vi "THzTime_SPEED_control_2_points_scan_TA_170302.vi"(1 "ESP300 Axis":i8=1, 2 "ESP300 Address":string="1", 4 "Lockin Address":string="12") -> ()   [LabVIEW 2010]
panel:
  out "Current Round":i32
  in  "ESP300 Axis 2":i8=2
  in  "Delay (ms)":u32=10000
  in  "# of Round":i8=10
  in  "Position 2":sgl=-33.5 min=-75 max=75 format="%#.3f"
  in  "Position 1":sgl=-35.0 min=-75 max=75 format="%#.3f"
  out "Y position":dbl=-149.05 format="%#.3p"
  out "X position":dbl=857.9 format="%#.3p"
  out "Power meter":dbl=68.74000000000001 format="%#.3p"
  in  "Save File Name":string
  in  "Launch server?":bool
  in  "Authorize?":bool=TRUE
  in  "CONEX-PSD9 Instrument Key 2":string="CONEX-PSD (A6ULD73M)"
  in  "Interdelay (ms)":dbl=20.0
  in  "pre delay(ms)":dbl=300.0
  out "Lock-in Y-Channel":dbl=2.5466e-11 format="%#.3p"
  out "Lock-in X-Channel":dbl=-5.457e-12 format="%#.3p"
  out "THz Time-domain Signal Wave":cluster{"x-axis":sgl[], "y-axis":dbl[]}(graph)={"x-axis"=[-3.0, -2.99, -2.98, -2.97, -2.96, -2.95, -2.94, -2.93, -2.92, -2.91, -2.9, -2.89, -2.88, -2.87, -2.86, -2.85, -2.84, -2.83, -2.82, -2.81, -2.8, -2.79, -2.78, -2.77, -2.76, -2.75, -2.74, -2.73, -2.72, -2.71, -2.7, -2.69, -2.68, -2.67, -2.66, -2.65, -2.64, -2.63, -2.6200001, -2.61, -2.6, -2.59, -2.58, -2.57, -2.56, -2.55, -2.54, -2.53, -2.52, -2.51, -2.5, -2.49, -2.48, -2.47, -2.46, -2.45, -2.44, -2.43, -2.42, -2.41, -2.4, -2.39, -2.38, -2.3700001, -2.3600001, -2.35, -2.34, -2.33, -2.32, -2.31, -2.3, -2.29, -2.28, -2.27, -2.26, -2.25, -2.24, -2.23, -2.22, -2.21, -2.2, -2.19, -2.18, -2.17, -2.16, -2.15, -2.14, -2.13, -2.1200001, -2.1100001, -2.1, -2.09, -2.08, -2.07, -2.06, -2.05, -2.04, -2.03, -2.02, -2.01, -2.0, -1.99, -1.98, -1.97, -1.96, -1.95, -1.94, -1.9300001, -1.9200001, -1.91, -1.9, -1.89, -1.88, -1.87, -1.86, -1.85, -1.84, -1.83, -1.82, -1.8100001, -1.8000001, -1.7900001, -1.78, -1.77, -1.76, -1.75, -1.74, -1.73, -1.72, -1.71, -1.7, -1.69, -1.6800001, -1.6700001, -1.6600001, -1.65, -1.64, -1.63, -1.62, -1.61, -1.6, -1.59, -1.58, -1.57, -1.5600001, -1.5500001, -1.5400001, -1.5300001, -1.52, -1.51, -1.5, -1.49, -1.48, -1.47, -1.46, -1.45, -1.44, -1.4300001, -1.4200001, -1.4100001, -1.4000001, -1.39, -1.38, -1.37, -1.36, -1.35, -1.34, -1.33, -1.32, -1.3100001, -1.3000001, -1.2900001, -1.2800001, -1.27, -1.26, -1.25, -1.24, -1.23, -1.22, -1.21, -1.2, -1.19, -1.1800001, -1.1700001, -1.1600001, -1.1500001, -1.14, -1.13, -1.12, -1.11, -1.1, -1.09, -1.08, -1.07, -1.0600001, -1.0500001, -1.0400001, -1.0300001, -1.0200001, -1.01, -1.0, -0.99000007], "y-axis"=[6.18461e-11, 6.18461e-11, 6.275559999999999e-11, 6.457460000000001e-11, 6.54841e-11, 6.63936e-11, 6.821255e-11, 7.00315e-11, 7.18505e-11, 7.36695e-11, 7.54885e-11, 7.6398e-11, 7.6398e-11, 7.8217e-11, 7.8217e-11, 7.8217e-11, 7.8217e-11, 7.8217e-11, 7.8217e-11, 7.8217e-11, 7.8217e-11, 7.8217e-11, 7.8217e-11, 7.8217e-11, 7.73075e-11, 7.6398e-11, 7.54885e-11, 7.4579e-11, 7.4579e-11, 7.4579e-11, 7.4579e-11, 7.4579e-11, 7.4579e-11, 7.4579e-11, 7.36695e-11, 7.276e-11, 7.276e-11, 7.276e-11, 7.18505e-11, 7.18505e-11, 7.276e-11, 7.18505e-11, 7.0941e-11, 7.0941e-11, 7.00315e-11, 6.9122e-11, 6.821255e-11, 6.63936e-11, 6.457460000000001e-11, 6.275559999999999e-11, 6.18461e-11, 6.18461e-11, 6.275559999999999e-11, 6.36651e-11, 6.63936e-11, 6.912205e-11, 7.275999999999999e-11, 7.6398e-11, 7.91265e-11, 8.09455e-11, 8.27645e-11, 8.3674e-11, 8.3674e-11, 8.3674e-11, 8.27645e-11, 8.09455e-11, 7.821699999999999e-11, 7.36695e-11, 6.821255e-11, 6.09366e-11, 5.54795e-11, 4.911295e-11, 4.2746500000000003e-11, 3.7289500000000003e-11, 3.2742e-11, 3.001355e-11, 2.7285e-11, 2.7285e-11, 2.819455e-11, 3.092305e-11, 3.4561000000000003e-11, 3.7289500000000003e-11, 3.9108499999999995e-11, 4.09275e-11, 4.45655e-11, 4.638445e-11, 5.00224e-11, 5.18414e-11, 5.36604e-11, 5.72985e-11, 5.82081e-11, 5.82081e-11, 5.82081e-11, 6.00271e-11, 6.09366e-11, 6.275559999999999e-11, 6.457460000000001e-11, 6.730305e-11, 7.00315e-11, 7.18505e-11, 7.36695e-11, 7.54885e-11, 7.6398e-11, 7.73075e-11, 7.8217e-11, 7.8217e-11, 7.8217e-11, 7.8217e-11, 7.8217e-11, 7.8217e-11, 7.8217e-11, 7.8217e-11, 7.8217e-11, 7.8217e-11, 7.8217e-11, 7.8217e-11, 7.91265e-11, 8.0036e-11, 8.0036e-11, 7.91265e-11, 7.8217e-11, 7.8217e-11, 7.8217e-11, 7.8217e-11, 7.91265e-11, 8.0036e-11, 8.0036e-11, 8.0036e-11, 8.09455e-11, 8.1855e-11, 8.09455e-11, 8.0036e-11, 7.91265e-11, 7.8217e-11, 7.8217e-11, 7.73075e-11, 7.54885e-11, 7.36695e-11, 7.18505e-11, 6.9122e-11, 6.73031e-11, 6.54841e-11, 6.457460000000001e-11, 6.36651e-11, 6.275559999999999e-11, 6.09366e-11, 6.00271e-11, 6.00271e-11, 6.00271e-11, 6.00271e-11, 6.09366e-11, 6.18461e-11, 6.18461e-11, 6.18461e-11, 6.275559999999999e-11, 6.36651e-11, 6.457460000000001e-11, 6.54841e-11, 6.457460000000001e-11, 6.36651e-11, 6.36651e-11, 6.36651e-11, 6.36651e-11, 6.36651e-11, 6.36651e-11, 6.36651e-11, 6.36651e-11, 6.36651e-11, 6.36651e-11, 6.36651e-11, 6.36651e-11, 6.36651e-11, 6.457460000000001e-11, 6.54841e-11, 6.457460000000001e-11, 6.457460000000001e-11, 6.54841e-11, 6.63936e-11, 6.73031e-11, 6.73031e-11, 6.9122e-11, 6.73031e-11, 6.821255e-11, 6.9122e-11, 6.9122e-11, 6.73031e-11, 6.821255e-11, 6.9122e-11, 6.9122e-11, 6.9122e-11, 6.9122e-11, 6.821255e-11, 6.73031e-11, 6.73031e-11, 6.73031e-11, 6.73031e-11, 6.73031e-11, 6.73031e-11, 6.63936e-11, 6.63936e-11, 6.54841e-11, 6.54841e-11]}
  in  "Autosave Directory for Long-term Average Scan":path=path "D:/taianh/Measurement Data"
  in  "OK Button":bool
  out "Data Type":string="outp ? 1"
  in  "Enum":enum16{"X", "Y", "Abs"}(ring)
  in  "Draw":bool
  in  "Exit Program":bool
  in  "Short term \nAverage#":i8=1
  in  "Step":sgl=0.005 min=0 max=10000 format="%.3f"
  in  "End Position":sgl=-10.5 min=-75 max=75 format="%#.3f"
  in  "Start Position":sgl=-6.0 min=-75 max=75 format="%#.3f"
  # "THz Experiment"
  # "Data"
  # "Auto-offset"
  # "Start Position (mm)"
  # "End Position (mm)"
  # "Step (mm)"
  # "Point Avg"
  # "Number of Round"
  # "Position 1 (mm)"
  # "Position 2 (mm)"
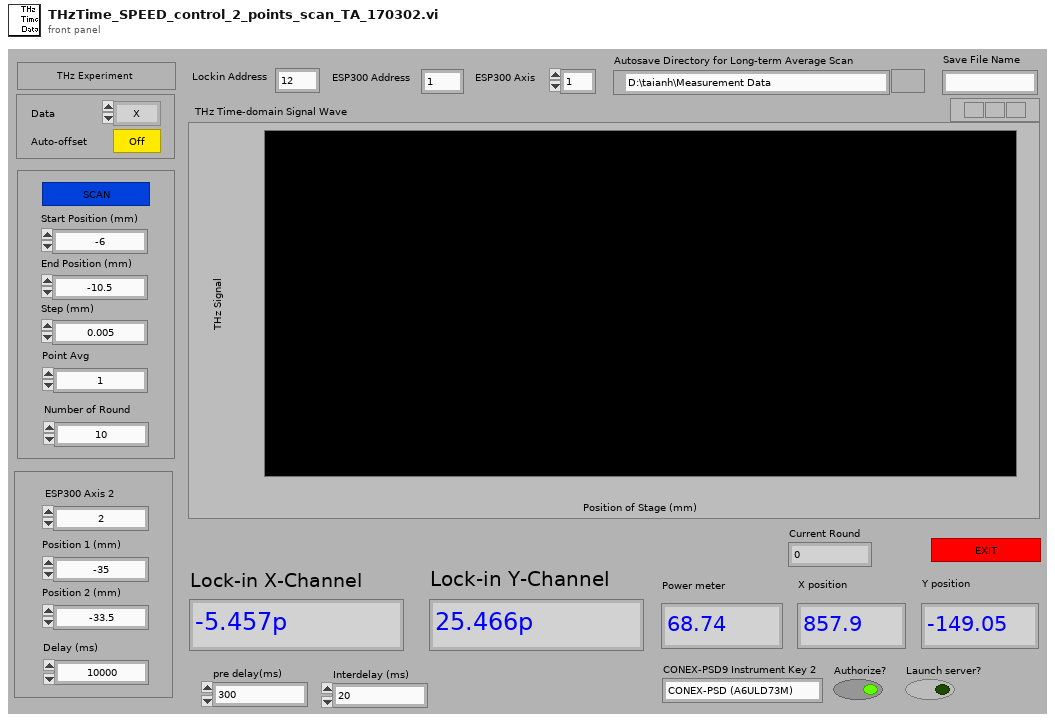
[diagram p1: front panel]
types:
  T1 = cluster{"ConexPSD Reference":refnum<k24>, "error out":errorcluster, "Component ID":i32}
  T2 = cluster{"Step Number":i32, "Step":sgl, "Start Position":sgl, "Time-out":i32, "Lockin Address":string, "Short term \nAverage#":i8, i32, "ESP300 Axis":i8, "Value":string, "pre delay(ms)":dbl, "Interdelay (ms)":dbl, "Autosave Directory for Long-term Average Scan":path, cluster{"ConexPSD Reference":refnum<k24>, "error out":errorcluster, "Component ID":i32}}
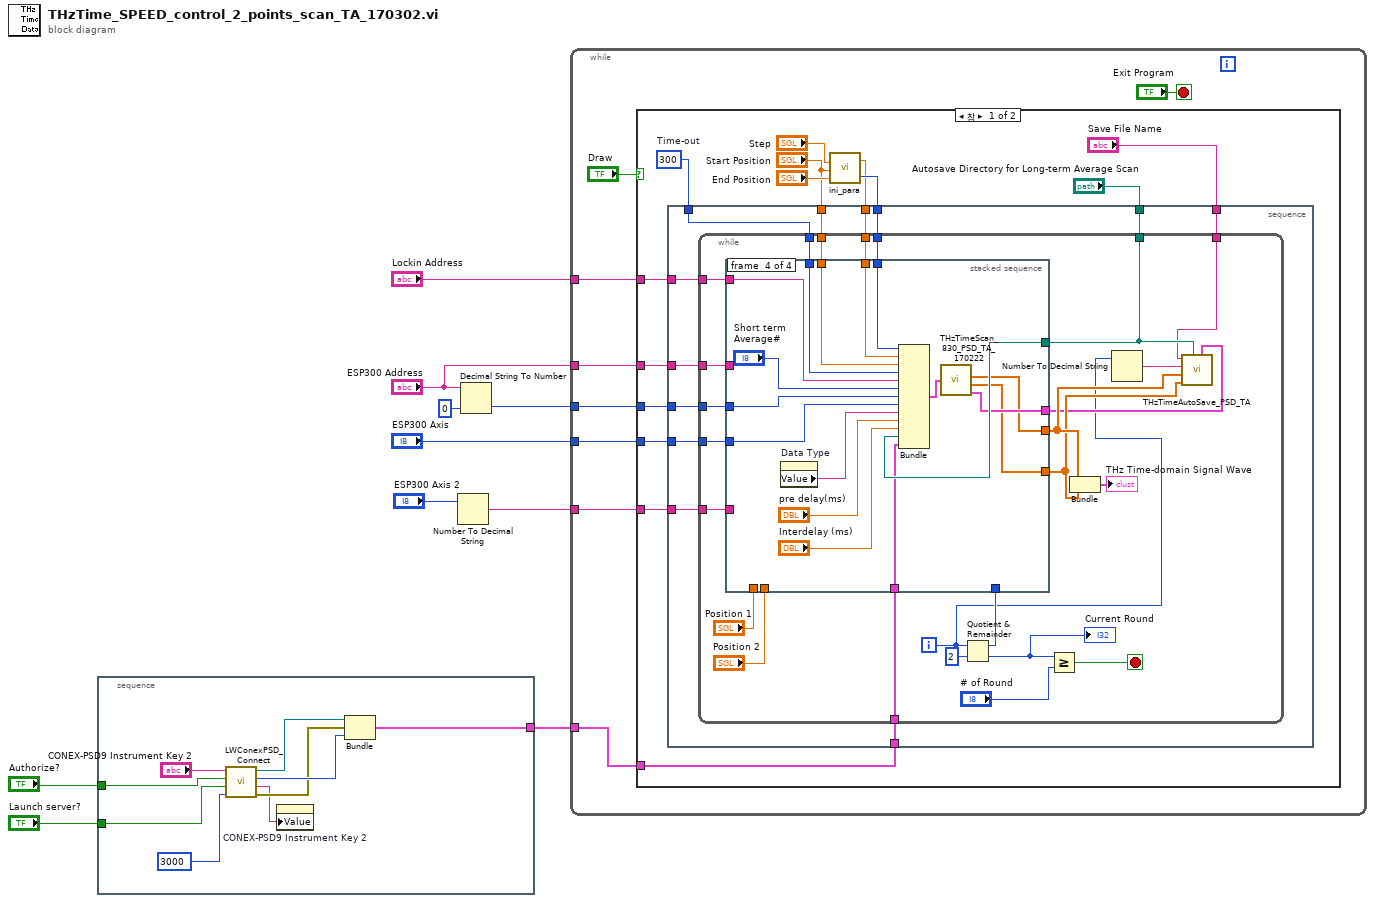
[diagram p0: block diagram]
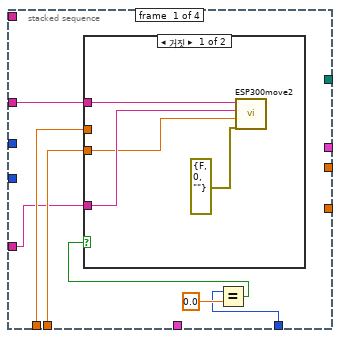
[diagram p2: hidden frame]
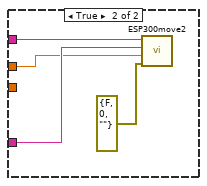
[diagram p3: hidden frame]
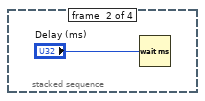
[diagram p4: hidden frame]
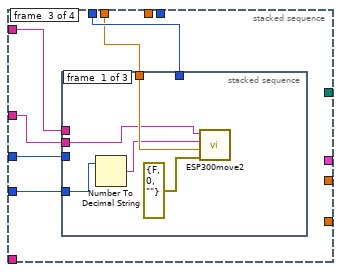
[diagram p5: hidden frame]
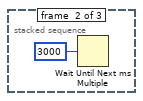
[diagram p6: hidden frame]
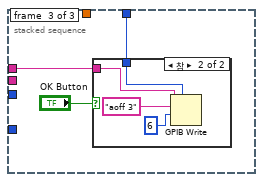
[diagram p7: hidden frame]
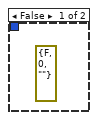
[diagram p8: hidden frame]
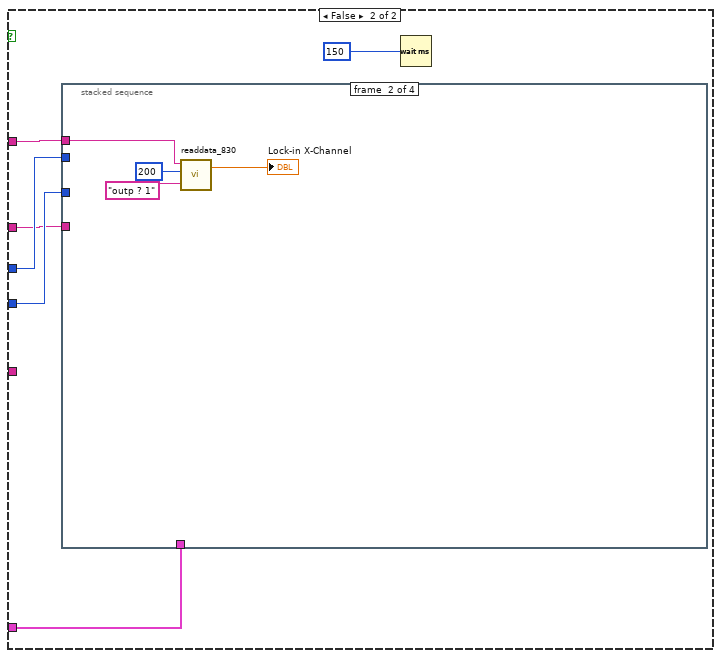
[diagram p9: hidden frame]
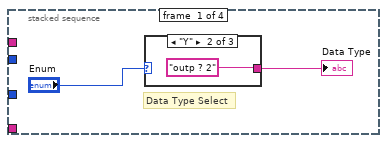
[diagram p10: hidden frame]
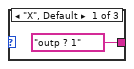
[diagram p11: hidden frame]
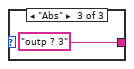
[diagram p12: hidden frame]
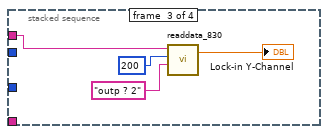
[diagram p13: hidden frame]
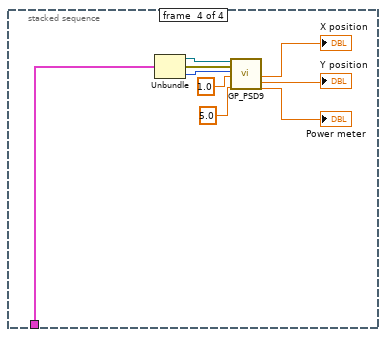
[diagram p14: hidden frame]
diagram:
  n1 = stacked-sequence {
    tunnel: "Authorize?" -> [w13]
    tunnel: [w12] -> w3
    tunnel: "Launch server?" -> [w11]
    frame #0 {
      n2 = call "LWConexPSD_Connect.vi"("DiscoverTimeout (10000 msec)"=3000, "Launch server? (True)"=w11, "Authorize? (True)"=w13, "Instrument Key"="CONEX-PSD9 Instrument Key 2") -> ("error out"=w17:errorcluster, "Instrument Key out"=w15:string, "Component ID"=w18:i32, "ConexPSD Reference"=w16:refnum<k24>)
      n3 = property on="CONEX-PSD9 Instrument Key 2" class="Str"("Value"=w15) -> ()  [unwired: 2 in, 2 out]
      n4 = Bundle("ConexPSD Reference"=w16, "error out"=w17, "Component ID"=w18) -> (w12:T1)  [unwired: 1 in]
    }
  }
  n5 = Number To Decimal String(number="ESP300 Axis 2") -> (decimal integer string=w1:string)  [unwired: 1 in]
  n6 = Decimal String To Number(string="ESP300 Address", default (0L)=0 ("default (0 I32)")) -> (number=w8:i32)  [unwired: 1 in, 1 out]
  n7 = while {
    tunnel: "ESP300 Axis" -> [w25]
    tunnel: "Lockin Address" -> [w24]
    tunnel: w8 -> [w23]
    tunnel: "ESP300 Address" -> [w22]
    tunnel: w3 -> [w21]
    tunnel: w1 -> [w20]
    stop <- "Exit Program" stop-if-true
    n8 = case shown="참" "Draw" {
      tunnel: w24 -> [w41 w134]
      tunnel: w25 -> [w40 w136]
      tunnel: w23 -> [w39 w135]
      tunnel: w22 -> [w31 w132]
      tunnel: w21 -> [w30 w131]
      tunnel: w20 -> [w28 _]
      frame True {
        w38 = 300  # Time-out
        n9 = call "ini_para.vi"("End Position"="End Position", "Start Position"="Start Position", "Step"="Step") -> ("Step Number"=w35:i32, "Step"=w34:sgl)
        n10 = stacked-sequence {
          tunnel: w41 -> [w53]
          tunnel: w38 -> [w52]
          tunnel: w40 -> [w51]
          tunnel: w39 -> [w50]
          tunnel: w35 -> [w48]
          tunnel: w34 -> [w46]
          tunnel: "Start Position" -> [w49]
          tunnel: "Autosave Directory for Long-term Average Scan" -> [w47]
          tunnel: w31 -> [w45]
          tunnel: w30 -> [w44]
          tunnel: "Save File Name" -> [w43]
          tunnel: w28 -> [w42]
          frame #0 {
            n11 = while {
              tunnel: w53 -> [w78]
              tunnel: w52 -> [w77]
              tunnel: w51 -> [w76]
              tunnel: w50 -> [w75]
              tunnel: w49 -> [w74]
              tunnel: w48 -> [w73]
              tunnel: w47 -> [w72]
              tunnel: w46 -> [w71]
              tunnel: w45 -> [w69]
              tunnel: w44 -> [w68]
              tunnel: w43 -> [w67]
              tunnel: w42 -> [w58]
              i -> [w55]
              stop <- w56 stop-if-true
              n12 = Quotient & Remainder(x=w55, y=2) -> (x-y*floor(x/y)=w61:i32, floor(x/y)=w54:i32)
              "Current Round" <- w54
              n13 = stacked-sequence {
                tunnel: w78 -> [_ _ w100 w126]
                tunnel: w77 -> [_ _ w99 w127]
                tunnel: w76 -> [_ _ w98 w123]
                tunnel: w75 -> [_ _ w97 w124]
                tunnel: w74 -> [_ _ w96 w128]
                tunnel: w71 -> [_ _ _ w129]
                tunnel: w73 -> [_ _ _ w130]
                tunnel: [_ _ _ w114] -> w70
                tunnel: [_ _ _ w115] -> w64
                tunnel: w69 -> [w81 _ w95 _]
                tunnel: w72 -> [_ _ _ w119]
                tunnel: w68 -> [_ _ _ w118]
                tunnel: [_ _ _ w116] -> w63
                tunnel: w61 -> [w79 _ _ _]
                tunnel: "Position 1" -> [w83 _ _ _]
                tunnel: "Position 2" -> [w82 _ _ _]
                tunnel: w58 -> [w80 _ _ _]
                frame #0 {
                  n14 = Equal?(x=w79, y=0.0) -> (x = y?=w84:bool)
                  n15 = case shown="거짓" w84 {
                    tunnel: w83 -> [_ w90]
                    tunnel: w82 -> [w86 _]
                    tunnel: w81 -> [w88 w93]
                    tunnel: w80 -> [w87 w92]
                    frame False {
                      n16 = call "ESP300move2.vi"("ESP300 Address"=w88, "ESP300 Channel"=w87, "Target"=w86, "error in (no error) 2"=errorcluster {"status"=FALSE, "code"=0, "source"=""}) -> ()  [unwired: 6 in, 1 out]
                    }
                    frame True {
                      n17 = call "ESP300move2.vi"("ESP300 Address"=w93, "ESP300 Channel"=w92, "Target"=w90, "error in (no error) 2"=errorcluster {"status"=FALSE, "code"=0, "source"=""}) -> ()  [unwired: 6 in, 1 out]
                    }
                  }
                }
                frame #1 {
                  n18 = Wait (ms)(milliseconds to wait="Delay (ms)") -> ()  [unwired: 1 out]
                }
                frame #2 {
                  n19 = stacked-sequence {
                    tunnel: w100 -> [_ _ w108]
                    tunnel: w99 -> [_ _ w107]
                    tunnel: w98 -> [w102 _ _]
                    tunnel: w97 -> [_ _ _]
                    tunnel: w96 -> [w105 _ _]
                    tunnel: w95 -> [w103 _ _]
                    frame #0 {
                      n20 = Number To Decimal String(number=w102) -> (decimal integer string=w101:string)  [unwired: 1 in]
                      n21 = call "ESP300move2.vi"("ESP300 Address"=w103, "ESP300 Channel"=w101, "Target"=w105, "error in (no error) 2"=errorcluster {"status"=FALSE, "code"=0, "source"=""}) -> ()  [unwired: 6 in, 1 out]
                    }
                    frame #1 {
                      n22 = Wait Until Next ms Multiple(millisecond multiple=3000) -> ()  [unwired: 1 out]
                    }
                    frame #2 {
                      n23 = case shown="참" "OK Button" {
                        tunnel: w108 -> [_ w113]
                        tunnel: w107 -> [_ w111]
                        frame False {
                          (unwired) errorcluster {"status"=FALSE, "code"=0, "source"=""} ("error in")
                        }
                        frame True {
                          n24 = GPIB Write(0:w113, 1:"aoff 3" ("data"), 2:i16 6 ("mode (0)"), 4:w111) -> ()  [unwired: 1 in, 2 out]
                        }
                      }
                    }
                  }
                }
                frame #3 {
                  n25 = property on="Data Type" class="Str"() -> ("Value"=w122:string)  [unwired: 2 in, 2 out]
                  n26 = Bundle("Step Number"=w130, "Step"=w129, "Start Position"=w128, "Time-out"=w127, "Lockin Address"=w126, "Short term \nAverage#"="Short term \nAverage#", w124, "ESP300 Axis"=w123, "Value"=w122, "pre delay(ms)"="pre delay(ms)", "Interdelay (ms)"="Interdelay (ms)", "Autosave Directory for Long-term Average Scan"=w119, w118) -> (w117:T2)  [unwired: 1 in]
                  n27 = call "THzTimeScan_830_PSD_TA_170222.vi"("input"=w117) -> ("x-axis"=w114:sgl[], "y-axis"=w115:dbl[], "ext. out"=w116:cluster{dbl[], dbl[], dbl[], dbl[], string[]})  [unwired: 1 out]
                }
              }
              n28 = Greater Or Equal?(x=w54, y="# of Round") -> (x >= y?=w56:bool)
              n29 = Bundle("x-axis"=w70, "y-axis"=w64) -> (→"THz Time-domain Signal Wave":cluster{"x-axis":sgl[], "y-axis":dbl[]})  [unwired: 1 in]
              n30 = Number To Decimal String(number=w55) -> (decimal integer string=w65:string)  [unwired: 1 in]
              n31 = call "THzTimeAutoSave_PSD_TA.vi"("ext. out"=w63, "Autosave Directory for Long-term Average Scan"=w72, "y-axis"=w64, "x-axis"=w70, "String"=w65, "SaveFile name"=w67) -> ()  [unwired: 4 in]
            }
          }
        }
      }
      frame False {
        n32 = stacked-sequence {
          tunnel: w136 -> [_ _ _ _]
          tunnel: w135 -> [_ _ _ _]
          tunnel: w134 -> [_ w145 w149 _]
          tunnel: w132 -> [_ _ _ _]
          tunnel: w131 -> [_ _ _ w150]
          frame #0 {
            # "Data Type Select"
            n33 = case shown="\"Y\"" "Enum" {
              tunnel: ["outp ? 1" "outp ? 2" "outp ? 3"] -> w138
              frame "X", Default {
              }
              frame "Y" {
              }
              frame "Abs" {
              }
            }
            "Data Type" <- w138
          }
          frame #1 {
            n34 = call "readdata_830.vi"("Command"="outp ? 1", "timeout"=200, "Lockin Address"=w145) -> ("Data"=→"Lock-in X-Channel":dbl)  [unwired: 1 in, 1 out]
          }
          frame #2 {
            n35 = call "readdata_830.vi"("Command"="outp ? 2", "timeout"=200, "Lockin Address"=w149) -> ("Data"=→"Lock-in Y-Channel":dbl)  [unwired: 1 in, 1 out]
          }
          frame #3 {
            n36 = Unbundle(w150) -> ("ConexPSD Reference"=w158:refnum<k24>, "error out"=w157:errorcluster, "Component ID"=w156:i32)
            n37 = call "GP_PSD9.vi"("ConexPSD Reference"=w158, "error out"=w157, "Component ID"=w156, "Adress"=1.0 ("shot average"), "shot average"=5.0) -> ("PositionX"=→"X position":dbl, "PositionY"=→"Y position":dbl, "LaserPower"=→"Power meter":dbl)  [unwired: 8 in, 4 out]
          }
        }
        n38 = Wait (ms)(milliseconds to wait=u32 150) -> ()  [unwired: 1 out]
      }
    }
  }
